vi "Binary_SpectroscopyFile-Read&ProcessTemplate.vi"() -> ()   [LabVIEW 2019]
doc: "Opens a binary file, then it loops over all spectroscopy experiment doing the following:\n\n - read spectroscopy data\n - determine I at a given voltage V by fitting a polynome to the data\n OR\n - determine dI/dV at a given voltage V by estimating the slope of a line fit\n\nThe (I @ V) or (dI/dV @ V) data is then displayed in a 3D display.\n\n- Nanonis Programming Interface -"
uses:
  <userlib>/Nanonis Prog Interface V5/Nanonis Prog Interface.lvlib
  <vilib>/Platform/NI_3dgraph.lvlib
panel:
  in  "Configuration":T1={"Mode"=enum."dI/dV @ V", "Bias voltage"=1.7, "Window width\n(# Points for fit)"=20, "Polynomial order\n(I/V @ V only)"=3}
  in  "3D Parametric Surface":refnum<k7>(container)
  out "error out":errorcluster
  in  "Binary Spectroscopy File":path
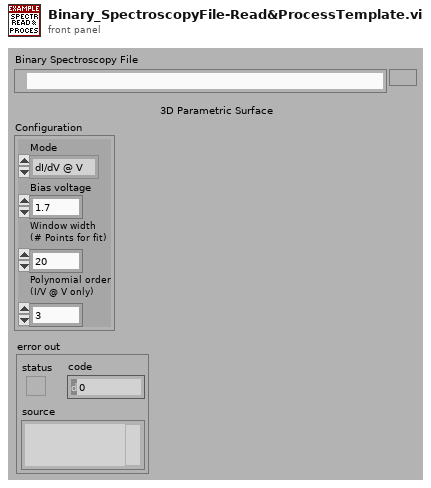
[diagram p1: front panel]
types:
  T1 = cluster{"Mode":enum16{"I @ V", "dI/dV @ V"}, "Bias voltage":sgl, "Window width\n(# Points for fit)":i32, "Polynomial order\n(I/V @ V only)":i32}
  T2 = typedef "Nanonis Prog Interface.lvlib/Binary_SpectroscopyFile-Config.ctl" = cluster{"Num Par":i32, "Exp size":i32, "Points":i32, "Grid Dim X":i32, "Grid Dim Y":i32, "Header size":i32, "Channels":string[], "Parameters":string[], "Sweep Signal":string, "Grid":cluster{"center X (m)":sgl, "center Y (m)":sgl, "width (m)":sgl, "height (m)":sgl, "angle (deg)":sgl}}
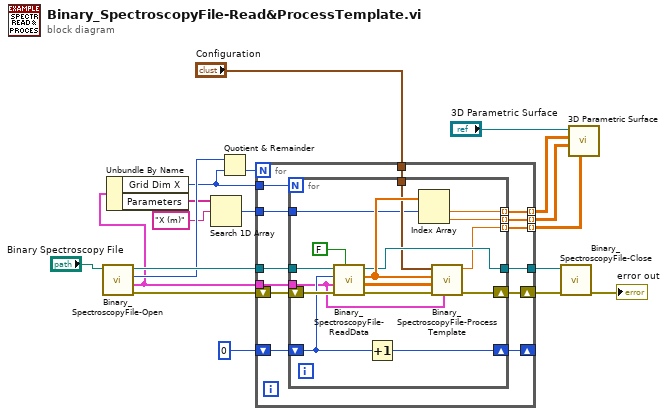
[diagram p0: block diagram]
diagram:
  n1 = call <userlib>:"Binary_SpectroscopyFile-Open.vi"("Binary Spectroscopy File"="Binary Spectroscopy File") -> ("error out"=w17:errorcluster, "Config"=w5:T2, "Number of Experiments"=w12:i32, "File ref"=w19:refnum<file>)  [unwired: 6 in, 1 out]
  n2 = Unbundle By Name(w5) -> ("Grid Dim X"=w4:i32, "Parameters"=w2:string[])
  n3 = Search 1D Array(1D array=w2, element="X (m)" ("string")) -> (index of element=w1:i32)  [unwired: 1 in]
  n4 = Quotient & Remainder(x=w12, y=w4) -> (floor(x/y)=w11:i32)  [unwired: 1 out]
  n5 = for {
    N: w11 -> [_]
    tunnel: w19 -> [w32]
    tunnel: w5 -> [w30]
    shift-right: [w29] -> w16
    shift-left: w17 -> [w31]
    tunnel: [w28] -> w15
    tunnel: w4 -> [w27]
    tunnel: [w26] -> w10 mode=indexing
    tunnel: [w25] -> w9 mode=indexing
    tunnel: [w24] -> w8 mode=indexing
    shift-right: [w22] -> _
    shift-left: 0 -> [w23]
    tunnel: "Configuration" -> [w21]
    tunnel: w1 -> [w20]
    n6 = for {
      N: w27 -> [_]
      tunnel: w32 -> [w48]
      tunnel: w30 -> [w34]
      tunnel: [w37] -> w28
      shift-right: [w38] -> w29
      shift-left: w31 -> [w47]
      tunnel: [w45] -> w26 mode=indexing
      tunnel: [w44] -> w25 mode=indexing
      tunnel: [w36] -> w24 mode=indexing
      shift-right: [w42] -> w22
      shift-left: w23 -> [w43]
      tunnel: w21 -> [w35]
      tunnel: w20 -> [w33]
      n7 = call <userlib>:"Binary_SpectroscopyFile-ReadData.vi"("Read Parameters only? (F)"=FALSE, "error in"=w47, "Config"=w34, "Experiment to read (Index)"=w43, "File ref In"=w48) -> ("error out"=w39:errorcluster, "data"=w40:sgl[][], "Parameter values"=w41:sgl[], "File ref Out"=w37:refnum<file>)  [unwired: 3 in]
      n8 = Increment(x=w43) -> (x+1=w42:i32)
      n9 = Index Array(array=w41, index #1=w33) -> (element #1=w45:sgl, element #2=w44:sgl)  [unwired: 1 in]
      n10 = call <userlib>:"Binary_SpectroscopyFile-ProcessTemplate.vi"("Config"=w34, "error in (no error)"=w39, "data"=w40, "Parameter values"=w41, "Configuration"=w35) -> ("error out"=w38:errorcluster, "Output value"=w36:sgl)  [unwired: 5 in]
    }
  }
  n11 = call <userlib>:"Binary_SpectroscopyFile-Close.vi"("error in"=w16, "File ref"=w15) -> ("error out"=→"error out":errorcluster)  [unwired: 9 in]
  n12 = call <vilib>:"3D Parametric Surface.vi"("z matrix"=w8, "y matrix"=w9, "x matrix"=w10, "3D graph"="3D Parametric Surface") -> ()  [unwired: 6 in, 2 out]
